vi "WT500 Example.vi"(8 "Error In":errorcluster) -> (0 "Error Out":errorcluster)   [LabVIEW 2016]
doc: "An example code of how to use Yokogawa's WT500 with LabVIEW. \nThe program initializes the instrument, reads the measurements, and then terminates the software connection to the instrument. \nAn error message also appears if any errors occur."
uses:
  Trunk/Utility/Type Definitions/UTILITY Power Data.ctl
panel:
  in  "stop":bool
  out "Output Array":dbl[](array[numeric])
  out "Data Array":string[][](array[string])
  out "Power Data Out":T1={"Current (A):Element 1"=236.2, "Current (A):Element 2"=17.749, "Power (W):Sigma"=4192.0, "Watt Hours (Wh):Sigma"=0.0, "Voltage (V):Element 2"=236.2, "Voltage (V):Element 1"=236.2, "Current Crest Factor:Element 1"=0.0, "Current Crest Factor:Element 2"=0.0, "Voltage Harmonic Content (%):Element 1"=0.0, "Voltage Harmonic Content (%):Element 2"=0.0, "Voltage Crest Factor:Element 1"=0.0, "Voltage Crest Factor:Element 2"=0.0, "Time:Element 1"=0.0, "Frequency (Hz):Element 1"=0.0, "Apparent Power (VA):Element 1"=0.0, "Apparent Power (VA):Element 2"=0.0, "Power Factor:Element 1"=0.0, "Power Factor:Element 2"=0.0, "Max Watt Hours"=0.0, "Voltage (V):Element 2 Avg"=0.0, "Voltage (V):Element 1 Avg"=0.0} {"Voltage (V):Element 1 Avg" format="%.3g"; "Voltage (V):Element 2 Avg" format="%.3g"; "Max Watt Hours" format="%.3g"; "Power Factor:Element 2" format="%.3g"; "Power Factor:Element 1" format="%.3g"; "Apparent Power (VA):Element 2" format="%.3g"; "Apparent Power (VA):Element 1" format="%.3g"; "Frequency (Hz):Element 1" format="%.3g"; "Time:Element 1" format="%.3g"; "Voltage Crest Factor:Element 2" format="%.3g"; "Voltage Crest Factor:Element 1" format="%.3g"; "Voltage Harmonic Content (%):Element 2" format="%.3g"; "Voltage Harmonic Content (%):Element 1" format="%.3g"; "Current Crest Factor:Element 2" format="%.3g"; "Current Crest Factor:Element 1" format="%.3g"; "Voltage (V):Element 1" format="%.3g"; "Voltage (V):Element 2" format="%.3g"; "Watt Hours (Wh):Sigma" format="%.3g"; "Power (W):Sigma" format="%.3g"; "Current (A):Element 2" format="%.3g"; "Current (A):Element 1" format="%.3g"}
  out "Label":string[](array[string])
  in  "I Range (7: 40A)":u16(ring)=7 items=["AUTO", "500 mA", "1 A", "2 A", "5 A", "10 A", "20 A", "40 A", "S-AUTO", "50 mV", "100 mV", "200 mV", "500 mV", "1 V", "2 V", "5 V", "10 V", "250 mA", "500 mA", "1 A", "2.5 A", "5 A", "10 A", "20 A", "25 mV", "50 mV", "100 mV", "250 mV", "500 mV", "1 V", "2.5 V", "5 V"]
  in  "V Range (8: 1000V)":u16(ring)=6 items=["AUTO", "15", "30", "60", "100", "150", "300", "600", "1000", "7.5", "15", "30", "50", "75", "150", "300", "500"]
  in  "VISA resource name":refnum<visa-resource-name>="WT500"
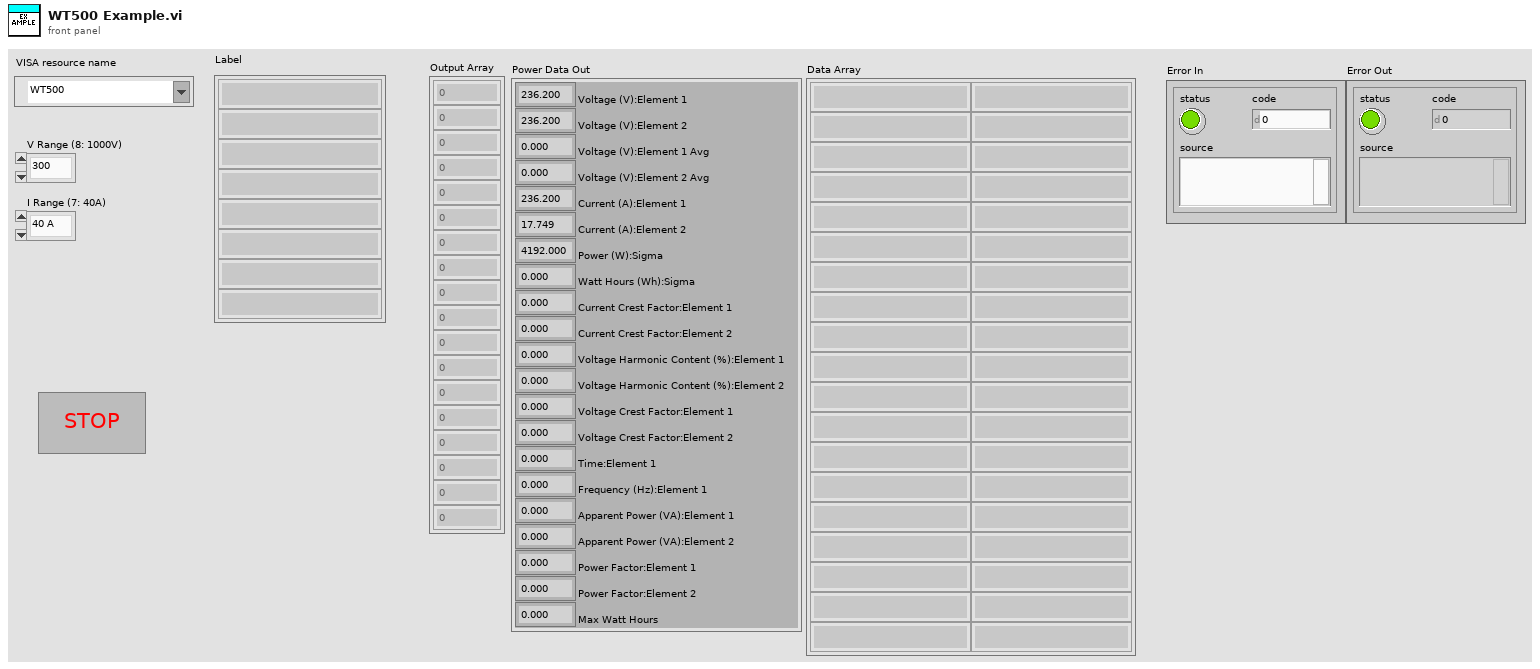
[diagram p1: front panel]
types:
  T1 = typedef "UTILITY Power Data.ctl" = cluster{"Current (A):Element 1":dbl, "Current (A):Element 2":dbl, "Power (W):Sigma":dbl, "Watt Hours (Wh):Sigma":dbl, "Voltage (V):Element 2":dbl, "Voltage (V):Element 1":dbl, "Current Crest Factor:Element 1":dbl, "Current Crest Factor:Element 2":dbl, "Voltage Harmonic Content (%):Element 1":dbl, "Voltage Harmonic Content (%):Element 2":dbl, "Voltage Crest Factor:Element 1":dbl, "Voltage Crest Factor:Element 2":dbl, "Time:Element 1":dbl, "Frequency (Hz):Element 1":dbl, "Apparent Power (VA):Element 1":dbl, "Apparent Power (VA):Element 2":dbl, "Power Factor:Element 1":dbl, "Power Factor:Element 2":dbl, "Max Watt Hours":dbl, "Voltage (V):Element 2 Avg":dbl, "Voltage (V):Element 1 Avg":dbl}
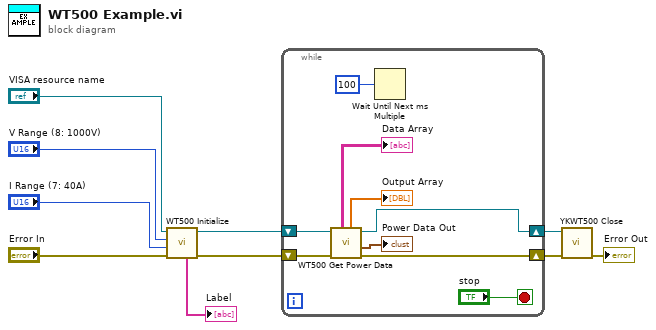
[diagram p0: block diagram]
diagram:
  n1 = call "WT500 Initialize.vi"("VISA resource name"="VISA resource name", "V Range (8: 1000V)"="V Range (8: 1000V)", "I Range (7: 40A)"="I Range (7: 40A)", "Error In (No Error) 2"="Error In") -> ("Label"=→"Label":string[], "VISA resource name out"=w8:refnum<visa-resource-name>, "Error Out"=w10:errorcluster)  [unwired: 4 in]
  n2 = while {
    shift-right: [w13] -> w3
    shift-left: w10 -> [w14]
    shift-right: [w18] -> w4
    shift-left: w8 -> [w19]
    stop <- "stop" stop-if-true
    n3 = call "WT500 Get Power Data.vi"("Error In"=w14, "VISA resource name"=w19) -> ("Error Out"=w13:errorcluster, "Power Data Out"=→"Power Data Out":T1, "VISA resource name out"=w18:refnum<visa-resource-name>, "Output Array"=→"Output Array":dbl[], "Data Array"=→"Data Array":string[][])  [unwired: 3 in, 1 out]
    n4 = Wait Until Next ms Multiple(millisecond multiple=u32 100) -> ()  [unwired: 1 out]
  }
  n5 = call "YKWT500 Close.vi"("error in (no error)"=w3, "VISA resource name"=w4) -> ("error out"=→"Error Out":errorcluster)  [unwired: 9 in]
